vi "MW_Freq_Set and Confirm.vi"(6 "Timout (5000ms, -1=never)":i32=5000, 7 "Tolerance Epsilon(10 Hz)":dbl=10.0 format="%#_13g", 8 "错误输入（无错误）":errorcluster, 10 "Set Frequency (Hz)":dbl, 11 "VISA引用句柄输入":refnum<visa-resource-name>) -> (0 "错误输出":errorcluster, 2 "Current Freq(Hz)":dbl, 3 "VISA引用句柄输出":refnum<visa-resource-name>)   [LabVIEW 2016, in "Microwave Source.lvlib"]
uses:
  Microwave Source.lvlib
panel:
  out "Used Time(ms)":u32
  out "Exectued times":i32
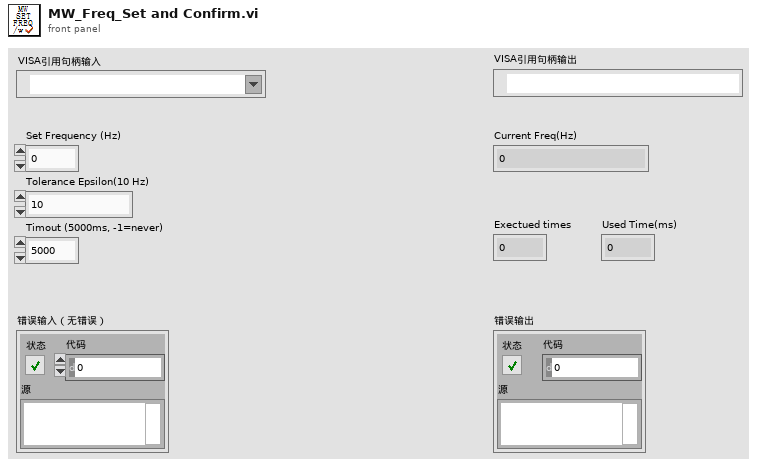
[diagram p1: front panel]
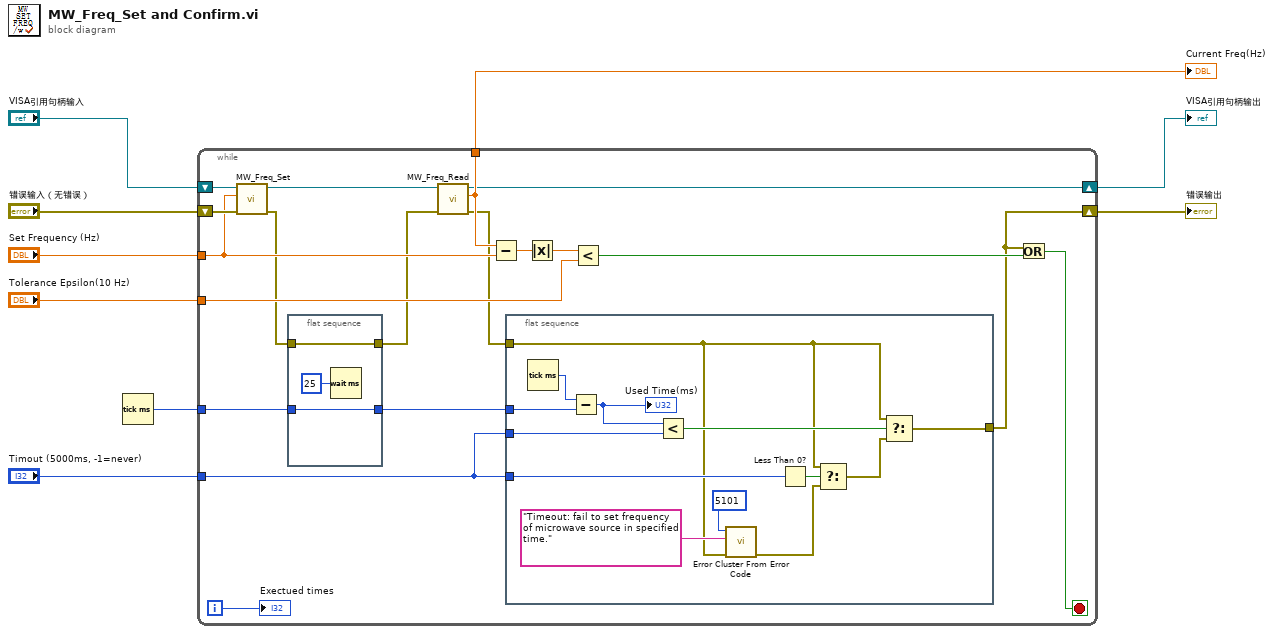
[diagram p0: block diagram]
diagram:
  n1 = Tick Count (ms)() -> (millisecond timer value=w2:u32)
  n2 = while {
    tunnel: [w25] -> w7
    tunnel: "Tolerance Epsilon(10 Hz)" -> [w22]
    tunnel: "Set Frequency (Hz)" -> [w20]
    shift-right: [w15] -> w3
    shift-left: "错误输入（无错误）" -> [w28]
    shift-right: [w19] -> w4
    shift-left: "VISA引用句柄输入" -> [w27]
    tunnel: w2 -> [w13]
    tunnel: "Timout (5000ms, -1=never)" -> [w12]
    i -> [w10]
    stop <- w11 stop-if-true
    n3 = call "MW_Freq_Set.vi"("错误输入（无错误）"=w28, "Set Frequency (Hz)"=w20, "VISA引用句柄输入"=w27) -> ("错误输出"=w18:errorcluster, "VISA引用句柄输出"=w21:refnum<visa-resource-name>)  [unwired: 6 in, 1 out]
    n4 = flat-sequence {
      tunnel: w18 -> [w43]
      tunnel: [w43] -> w17
      tunnel: [w42] -> w14
      tunnel: w13 -> [w42]
      frame #0 {
        n5 = Wait (ms)(milliseconds to wait=u32 25) -> ()  [unwired: 1 out]
      }
    }
    n6 = call "MW_Freq_Read.vi"("错误输入（无错误）"=w17, "VISA引用句柄输入"=w21) -> ("错误输出"=w16:errorcluster, "Freq(GHz)"=w25:dbl, "VISA引用句柄输出"=w19:refnum<visa-resource-name>)  [unwired: 6 in, 1 out]
    n7 = Subtract(x=w25, y=w20) -> (x-y=w26:dbl)
    n8 = flat-sequence {
      tunnel: w16 -> [w32]
      tunnel: [w29] -> w15
      tunnel: w14 -> [w40]
      tunnel: w12 -> [w38]
      tunnel: w12 -> [w34]
      frame #0 {
        n9 = Tick Count (ms)() -> (millisecond timer value=w41:u32)
        n10 = Subtract(x=w41, y=w40) -> (x-y=w39:u32)
        "Used Time(ms)" <- w39
        n11 = Less?(x=w39, y=w38) -> (x < y?=w37:bool)
        n12 = call <vilib>:"Error Cluster From Error Code.vi"("error in (no error)"=w32, "error message (\"\")"="Timeout: fail to set frequency of microwave source in specified time." ("error message (\"\")"), "error code (0)"=5101) -> ("error out"=w31:errorcluster)  [unwired: 6 in]
        n13 = Less Than 0?(x=w34) -> (x < 0?=w33:bool)
        n14 = Select(t=w32, s=w33, f=w31) -> (s? t:f=w30:errorcluster)
        n15 = Select(t=w32, s=w37, f=w30) -> (s? t:f=w29:errorcluster)
      }
    }
    n16 = Absolute Value(x=w26) -> (abs(x)=w23:dbl)
    n17 = Less?(x=w23, y=w22) -> (x < y?=w24:bool)
    n18 = Or(x=w15, y=w24) -> (x .or. y?=w11:bool)
    "Exectued times" <- w10
  }
  "错误输出" <- w3
  "VISA引用句柄输出" <- w4
  "Current Freq(Hz)" <- w7
